vi "Configure.vi"(8 "error in (no error)":errorcluster, 11 "GRMActor in":refnum<class "FlatFieldUI.lvclass">) -> (0 "error out":errorcluster, 3 "GRMActor out":refnum<class "FlatFieldUI.lvclass">)   [LabVIEW 2020, in "FlatField.lvlib" / "FlatFieldUI.lvlib" / "FlatFieldUI.lvclass"]
uses:
  FlatFieldUI/FlatFieldUI.lvclass
  Hardware Abstraction Layer/Component/GenericActor/GenericActor/GenericController.lvclass
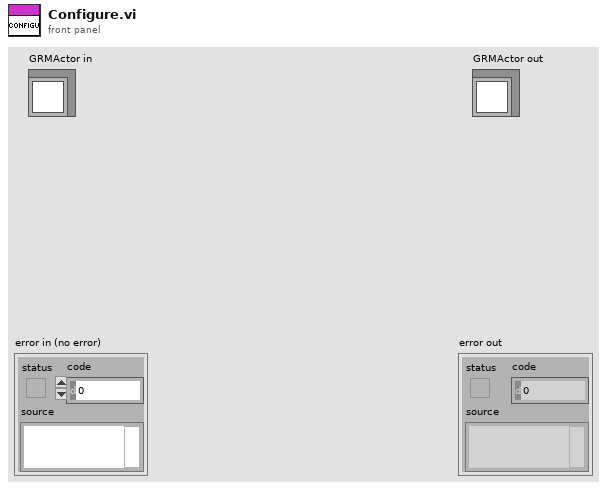
[diagram p1: front panel]
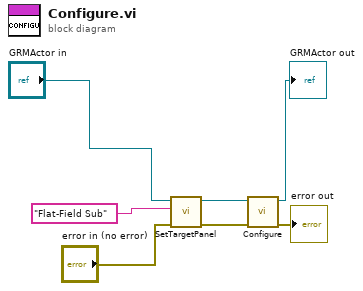
[diagram p0: block diagram]
diagram:
  n1 = call-dynamic "SetTargetPanel.vi"("error in (no error)"="error in (no error)", "TargetPanel"="Flat-Field Sub", "GRMActor in"="GRMActor in") -> ("error out"=w5:errorcluster, "GRMActor out"=w4:refnum<class "FlatFieldUI.lvclass">)  [unwired: 7 in]
  n2 = call-parent "Configure.vi"("error in (no error)"=w5, "GRMActor in"=w4) -> ("error out"=→"error out":errorcluster, "GRMActor out"=→"GRMActor out":refnum<class "FlatFieldUI.lvclass">)  [unwired: 8 in]
